vi "Get Time from ClockID.vi"(8 "error in (no error)":errorcluster, 9 "Reset Clock T0":bool, 11 "CIFCorePlugin in":refnum<class "CIFCorePlugin.lvclass">) -> (0 "error out":errorcluster, 1 "Clock T0 changed":bool, 2 "ClockID Time (ns)":u64, 3 "CIFCorePlugin out":refnum<class "CIFCorePlugin.lvclass">)   [LabVIEW 2021, in "CIFCorePlugin.lvclass"]
uses:
  CIFCorePlugin.lvclass
  CIFCorePlugin.lvclass/CIFCorePlugin.ctl
  CIFUtilities/CIFClocks/Time Conversion/LabVIEW Time to UTC Time.vi
  CIFUtilities/CIFClocks/SubVIs/Add Error.vi
  CIFUtilities/CIFClocks/CIFClocks.lvlib
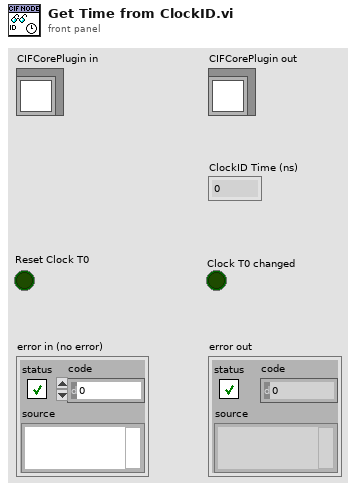
[diagram p1: front panel]
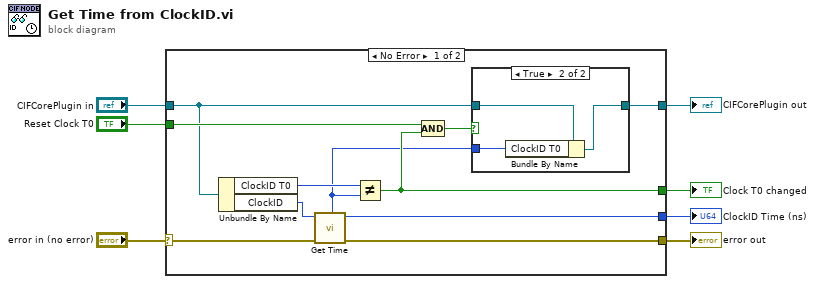
[diagram p0: block diagram]
diagram:
  n1 = case shown="No Error" "error in (no error)" {
    selector: "error in (no error)" -> [w16 w23]
    tunnel: [w17 w23] -> w4
    tunnel: [w8 w24] -> w6
    tunnel: "CIFCorePlugin in" -> [w9 w24]
    tunnel: [w18 _] -> w3
    tunnel: [w12 _] -> w2
    tunnel: "Reset Clock T0" -> [w13 _]
    frame No Error {
      n2 = Unbundle By Name(w9) -> ("ClockID T0"=w14:u64, "ClockID"=w15:u8)
      n3 = call "Get Time.vi"("error in (no error)"=w16, "ClockID"=w15) -> ("error out"=w17:errorcluster, "Time (ns)"=w18:u64, "T0"=w10:u64)  [unwired: 7 in]
      n4 = Not Equal?(x=w14, y=w10) -> (x != y?=w12:bool)
      n5 = Compound Arithmetic op=AND(w13, w12) -> (w11:bool)
      n6 = case shown="True" w11 {
        tunnel: w10 -> [_ w21]
        tunnel: w9 -> [w19 w22]
        tunnel: [w19 w20] -> w8
        frame False {
        }
        frame True {
          n7 = Bundle By Name(cluster=w22, "ClockID T0"=w21) -> (w20:refnum<class "CIFCorePlugin.lvclass">)
        }
      }
    }
    frame Error {
    }
  }
  "error out" <- w4
  "CIFCorePlugin out" <- w6
  "ClockID Time (ns)" <- w3
  "Clock T0 changed" <- w2
